vi "checkout.vi"(0 "HGF_Reference":refnum<class "HGF_Reference.lvclass">, 3 "timeout in ms (-1)":i32=-1, 5 "error in (no error)":errorcluster) -> (14 "dup HGF_Reference":refnum<class "HGF_Reference.lvclass">, 16 "HB_Simple":refnum<class "HB_Simple.lvclass">, 17 "got object?":bool, 19 "error out":errorcluster)   [LabVIEW 2009, in "HB_BaseClass_Examples.lvlib" / "HB_Simple.lvclass"]
doc: "Check out the referenced Object.\n\n<B>Attention:</B> Error in is ignored, but forwarded.\nDo not forget to check in again, if you have got the object."
uses:
  HB_Simple.lvclass
  lib.lib/HGF_LVC/HGF_BaseClasses/HGF_Reference/HGF_Reference.lvclass
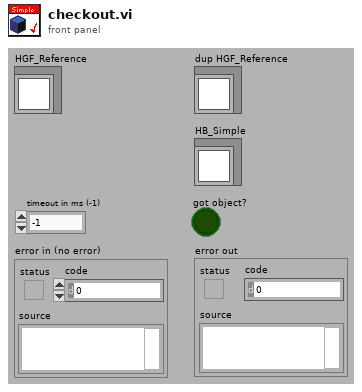
[diagram p1: front panel]
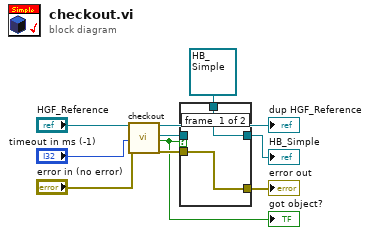
[diagram p0: block diagram]
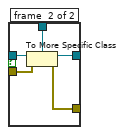
[diagram p2: hidden frame]
diagram:
  n1 = call "checkout.vi"("HGF_Reference"="HGF_Reference", "timeout in ms (-1)"="timeout in ms (-1)", "error in (no error)"="error in (no error)") -> ("dup HGF_Reference"=→"dup HGF_Reference":refnum<class "HGF_Reference.lvclass">, "Object"=w7:refnum<class>, "got object?"=w1:bool, "error out"=w4:errorcluster)  [unwired: 13 out]
  "got object?" <- w1
  n2 = case shown="True" w1 {
    tunnel: w7 -> [_ w17]
    tunnel: refnum<class "HB_Simple.lvclass"> refnum ("HB_HGF_Test.lvlib:HB_Simple.lvclass") -> [w12 w16]
    tunnel: w4 -> [w11 w15]
    tunnel: [w11 w14] -> w3
    tunnel: [w12 w13] -> w2
    frame #0 {
    }
    frame #1 {
      n3 = To More Specific Class(target class=w16, reference=w17, error in=w15) -> (specific class reference=w13:refnum<class "HB_Simple.lvclass">, error out=w14:errorcluster)
    }
  }
  "HB_Simple" <- w2
  "error out" <- w3
